vi "LaunchBall.vi"(8 "error in (no error)":errorcluster) -> (0 "error out":errorcluster)   [LabVIEW 2013]
uses:
  <vilib>/Rock Robotics/WPI/CAN/Jaguar/SubVIs/WPI_CANJaguar_StatusSelect.ctl
  Robot Global Data.vi
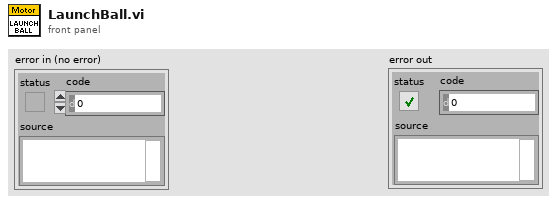
[diagram p1: front panel]
types:
  T1 = typedef "WPI_CANJaguar_StatusSelect.ctl" = enum16{"Output Percent VBus", "Output Voltage", "Bus Voltage", "Current", "Temperature", "Position", "Speed", "Limit Switches", "Faults", "Fault Counters", "Power Cycle"}
  T2 = typedef "WPI_MotorControlDeviceRef.ctl" = cluster{"DeviceStatus":errorcluster, "Type":enum16{"PWM", "CAN"}, "PWM":cluster{"Digital Module":T3, "PWM Channel":T4, "DeadBand":T5}, "CAN":cluster{"Device Number":u8, "Control Mode":T6, "Semaphore":T7, "Max Vout":dbl}, "Invert":bool, "TransformRef":T8, "InvTransformRef":T8}
  T3 = typedef "FPGA_TypedefDigitalModule.ctl" = enum16{"Digital Module 1", "Digital Module 2"}
  T4 = typedef "FPGA_DIOPWMChannel.ctl" = enum8{"PWM 1", "PWM 2", "PWM 3", "PWM 4", "PWM 5", "PWM 6", "PWM 7", "PWM 8", "PWM 9", "PWM 10", "Invalid"}
  T5 = typedef "WPI_PWMDeadband.ctl" = cluster{"Name":string, "maxPositivePwm":i32, "minPositivePwm":i32, "centerPwm":i32, "maxNegativePwm":i32, "minNegativePwm":i32, "angularRange":u16}
  T6 = typedef "WPI_CANJaguar_ControlMode.ctl" = enum8{"Percent VBus", "Current", "Speed", "Position", "Voltage"}
  T7 = typedef "Semaphore RefNum" = refnum<k1>
  T8 = typedef "WPI_PWMTransform_ConPane.ctl" = refnum<vi>
  T9 = typedef "WPI_CANJaguar_Status.ctl" = cluster{"Output Percent VBus":dbl, "Output Voltage":dbl, "Bus Voltage":dbl, "Current":dbl, "Temperature":dbl, "Position":dbl, "Speed":dbl, "Limits":cluster{"Forward Limit":bool, "Reverse Limit":bool, "Forward Soft Limit":bool, "Reverse Soft Limit":bool, "Sticky Forward Limit":bool, "Sticky Reverse Limit":bool, "Sticky Forward Soft Limit":bool, "Sticky Reverse Soft Limit":bool}, "Faults":cluster{"Current Fault":bool, "Temperature Fault":bool, "Bus Voltage Fault":bool, "Gate Driver Fault":bool, "Comm Fault":bool}, "Fault Counters":cluster{"Current Faults":u8, "Temperature Faults":u8, "Bus Voltage Faults":u8, "Gate Driver Faults":u8, "Comm Faults":u8, "CAN Status":u8, "CAN RX Errors":u8, "CAN TX Errors":u8}, "Power Cycle":bool}
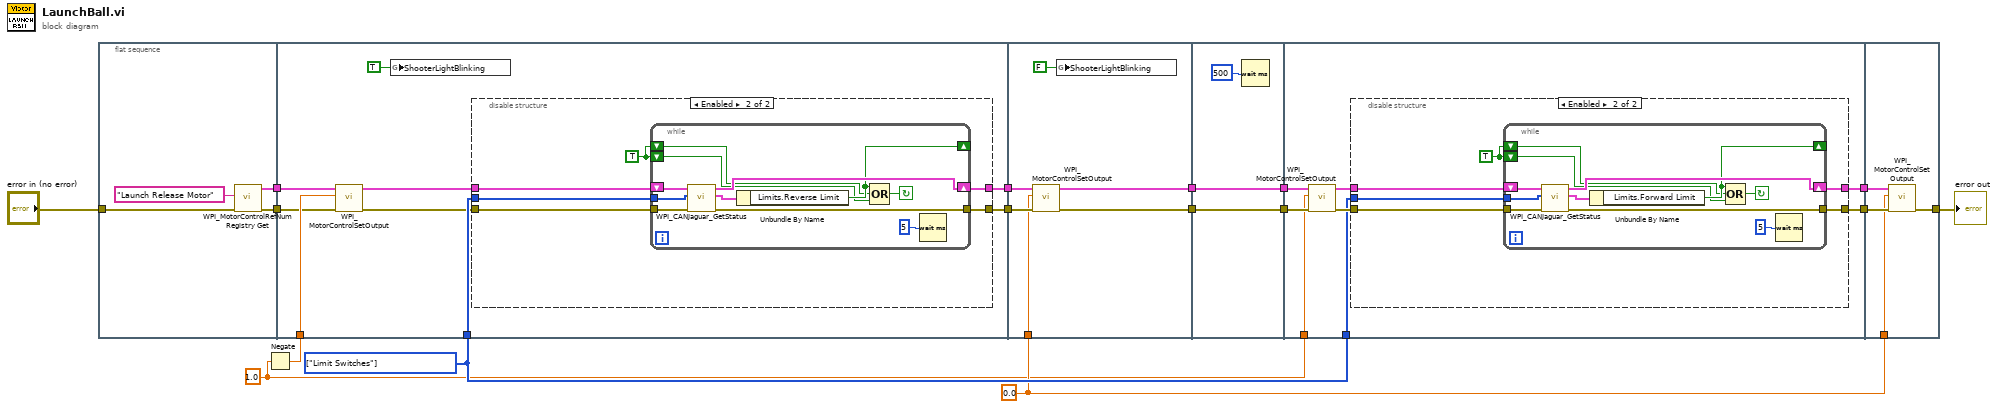
[diagram p0: block diagram]
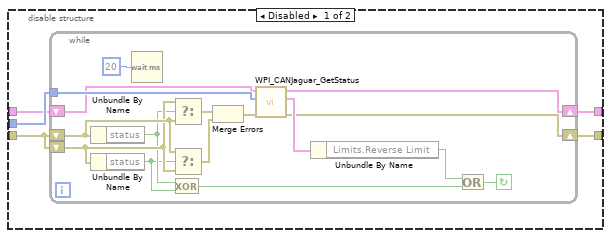
[diagram p2: hidden frame]
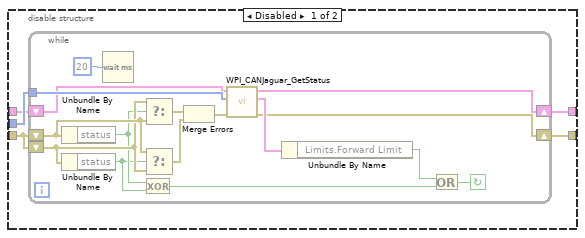
[diagram p3: hidden frame]
diagram:
  w4 = 0.0 ("Output")
  w3 = 1.0 ("Output")
  w10 = T1[] [enum."Limit Switches"] items=["Output Percent VBus", "Output Voltage", "Bus Voltage", "Current", "Temperature", "Position", "Speed", "Limit Switches", "Faults", "Fault Counters", "Power Cycle"] ("Status Select")
  n1 = flat-sequence {
    tunnel: "error in (no error)" -> [w20]
    tunnel: [w18] -> w16
    tunnel: [w17] -> w15
    tunnel: w16 -> [w25]
    tunnel: w15 -> [w24]
    tunnel: [w28] -> w14
    tunnel: [w29] -> w13
    tunnel: w10 -> [w27]
    tunnel: w5 -> [w26]
    tunnel: [w73] -> w9
    tunnel: [w72] -> w7
    tunnel: w13 -> [w70]
    tunnel: w14 -> [w71]
    tunnel: w4 -> [w69]
    tunnel: w9 -> [w76]
    tunnel: [w76] -> w8
    tunnel: w7 -> [w75]
    tunnel: [w75] -> w6
    tunnel: w8 -> [w84]
    tunnel: w6 -> [w83]
    tunnel: w10 -> [w79]
    tunnel: w3 -> [w82]
    tunnel: [w77] -> w2
    tunnel: [w78] -> w1
    tunnel: [w124] -> w12
    tunnel: w4 -> [w123]
    tunnel: w2 -> [w125]
    tunnel: w1 -> [w126]
    frame #0 {
      n2 = call <vilib>:"WPI_MotorControlRefNum Registry Get.vi"("error in (no error)"=w20, "refnum name"="Launch Release Motor") -> ("error out"=w17:errorcluster, "MotorControlDevRef"=w18:T2)  [unwired: 8 in]
    }
    frame #1 {
      n3 = call <vilib>:"WPI_MotorControlSetOutput.vi"("error in (no error)"=w24, "Output"=w26, "MotorControlDevRef"=w25) -> ("error out"=w22:errorcluster, "MotorControlDevRef"=w23:T2)  [unwired: 6 in, 1 out]
      n4 = global write "Robot Global Data.vi" "ShooterLightBlinking"(TRUE ("ShooterLightBlinking")) -> ()
      n5 = disable-structure shown="Enabled" {
        disable-tunnel: [w34 w52] -> w29
        disable-tunnel: [w33 w55] -> w28
        disable-tunnel: w27 -> [w32 w56]
        disable-tunnel: w23 -> [w31 w54]
        disable-tunnel: w22 -> [w30 w53]
        frame Disabled {
          n6 = while {
            shift-right: [w48] -> w34
            shift-left: w30 -> [w44]
            shift-right: [w47] -> w33
            shift-left: w31 -> [w45]
            tunnel: w32 -> [w46]
            shift-left: w30 -> [w43]
            stop <- w35 continue-if-true
            n7 = Unbundle By Name(w44) -> ("status"=w37:bool)
            n8 = Unbundle By Name(w43) -> ("status"=w36:bool)
            n9 = Wait (ms)(milliseconds to wait=u32 20) -> ()  [unwired: 1 out]
            n10 = Exclusive Or(1:w36, 2:w37) -> (0:w38:bool)
            n11 = Select(t=w43, s=w37, f=w44) -> (s? t:f=w41:errorcluster)
            n12 = Select(t=w44, s=w36, f=w43) -> (s? t:f=w42:errorcluster)
            n13 = Merge Errors(w41, w42) -> (w40:errorcluster)
            n14 = call <vilib>:"WPI_CANJaguar_GetStatus.vi"("error in (no error)"=w40, "Status Select"=w46, "CAN Jaguar Ref"=w45) -> ("error out"=w48:errorcluster, "Status"=w50:T9, "CAN Jaguar Ref Out"=w47:T2)  [unwired: 6 in]
            n15 = Unbundle By Name(w50) -> ("Limits.Reverse Limit"=w39:bool)
            n16 = Or(x=w39, y=w38) -> (x .or. y?=w35:bool)
          }
        }
        frame Enabled {
          w51 = TRUE
          n17 = while {
            shift-right: [w65] -> w55
            shift-left: w54 -> [w63]
            tunnel: w56 -> [w64]
            tunnel: w53 -> [w62]
            tunnel: [w61] -> w52
            shift-right: [w60] -> _
            shift-left: w51 -> [w59]
            shift-left: w51 -> [w58]
            stop <- w57 continue-if-true
            n18 = call <vilib>:"WPI_CANJaguar_GetStatus.vi"("error in (no error)"=w62, "Status Select"=w64, "CAN Jaguar Ref"=w63) -> ("error out"=w61:errorcluster, "Status"=w67:T9, "CAN Jaguar Ref Out"=w65:T2)  [unwired: 6 in]
            n19 = Unbundle By Name(w67) -> ("Limits.Reverse Limit"=w60:bool)
            n20 = Compound Arithmetic op=OR(w60, w59, w58) -> (w57:bool)
            n21 = Wait (ms)(milliseconds to wait=u32 5) -> ()  [unwired: 1 out]
          }
        }
      }
    }
    frame #2 {
      n22 = call <vilib>:"WPI_MotorControlSetOutput.vi"("error in (no error)"=w70, "Output"=w69, "MotorControlDevRef"=w71) -> ("error out"=w72:errorcluster, "MotorControlDevRef"=w73:T2)  [unwired: 6 in, 1 out]
      n23 = global write "Robot Global Data.vi" "ShooterLightBlinking"(FALSE) -> ()
    }
    frame #3 {
      n24 = Wait (ms)(milliseconds to wait=u32 500) -> ()  [unwired: 1 out]
    }
    frame #4 {
      n25 = call <vilib>:"WPI_MotorControlSetOutput.vi"("error in (no error)"=w83, "Output"=w82, "MotorControlDevRef"=w84) -> ("error out"=w81:errorcluster, "MotorControlDevRef"=w80:T2)  [unwired: 6 in, 1 out]
      n26 = disable-structure shown="Enabled" {
        disable-tunnel: [w89 w107] -> w78
        disable-tunnel: [w88 w106] -> w77
        disable-tunnel: w79 -> [w87 w109]
        disable-tunnel: w80 -> [w86 w110]
        disable-tunnel: w81 -> [w85 w108]
        frame Disabled {
          n27 = while {
            shift-right: [w103] -> w89
            shift-left: w85 -> [w99]
            shift-right: [w102] -> w88
            shift-left: w86 -> [w100]
            tunnel: w87 -> [w101]
            shift-left: w85 -> [w98]
            stop <- w90 continue-if-true
            n28 = Unbundle By Name(w99) -> ("status"=w92:bool)
            n29 = Unbundle By Name(w98) -> ("status"=w91:bool)
            n30 = Wait (ms)(milliseconds to wait=u32 20) -> ()  [unwired: 1 out]
            n31 = Exclusive Or(1:w91, 2:w92) -> (0:w93:bool)
            n32 = Select(t=w98, s=w92, f=w99) -> (s? t:f=w96:errorcluster)
            n33 = Select(t=w99, s=w91, f=w98) -> (s? t:f=w97:errorcluster)
            n34 = Merge Errors(w96, w97) -> (w95:errorcluster)
            n35 = call <vilib>:"WPI_CANJaguar_GetStatus.vi"("error in (no error)"=w95, "Status Select"=w101, "CAN Jaguar Ref"=w100) -> ("error out"=w103:errorcluster, "Status"=w105:T9, "CAN Jaguar Ref Out"=w102:T2)  [unwired: 6 in]
            n36 = Unbundle By Name(w105) -> ("Limits.Forward Limit"=w94:bool)
            n37 = Or(x=w94, y=w93) -> (x .or. y?=w90:bool)
          }
        }
        frame Enabled {
          w111 = TRUE
          n38 = while {
            shift-right: [w120] -> w106
            shift-left: w110 -> [w118]
            tunnel: w109 -> [w119]
            tunnel: w108 -> [w117]
            tunnel: [w116] -> w107
            shift-right: [w115] -> _
            shift-left: w111 -> [w114]
            shift-left: w111 -> [w113]
            stop <- w112 continue-if-true
            n39 = call <vilib>:"WPI_CANJaguar_GetStatus.vi"("error in (no error)"=w117, "Status Select"=w119, "CAN Jaguar Ref"=w118) -> ("error out"=w116:errorcluster, "Status"=w122:T9, "CAN Jaguar Ref Out"=w120:T2)  [unwired: 6 in]
            n40 = Unbundle By Name(w122) -> ("Limits.Forward Limit"=w115:bool)
            n41 = Compound Arithmetic op=OR(w115, w114, w113) -> (w112:bool)
            n42 = Wait (ms)(milliseconds to wait=u32 5) -> ()  [unwired: 1 out]
          }
        }
      }
    }
    frame #5 {
      n43 = call <vilib>:"WPI_MotorControlSetOutput.vi"("error in (no error)"=w126, "Output"=w123, "MotorControlDevRef"=w125) -> ("error out"=w124:errorcluster)  [unwired: 6 in, 2 out]
    }
  }
  n44 = Negate(x=w3) -> (-x=w5:dbl)
  "error out" <- w12
